vi "0006_FireAtSpecificTimeOnSpecificWeekdays.vi"(8 "error in (no error)":errorcluster) -> (0 "error out":errorcluster)   [LabVIEW 2013]
uses:
  <vilib>/addons/_JKI Toolkits/Caraya/classes/Assert/Assert True.vi
  <vilib>/addons/_JKI Toolkits/Caraya/classes/Test/Test.lvclass
  <vilib>/addons/_JKI Toolkits/Caraya/classes/Assert/Assert.lvclass
  source/openCron.lvlib
panel:
  out "after weekend":timestamp
  out "Occurences":timestamp[](array[timestamp])
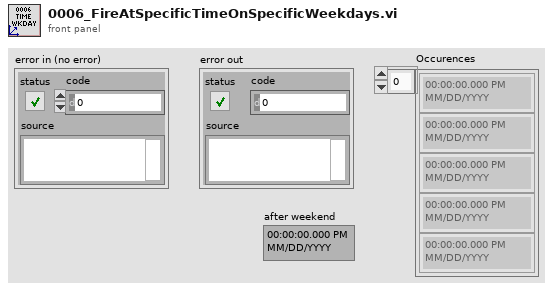
[diagram p1: front panel]
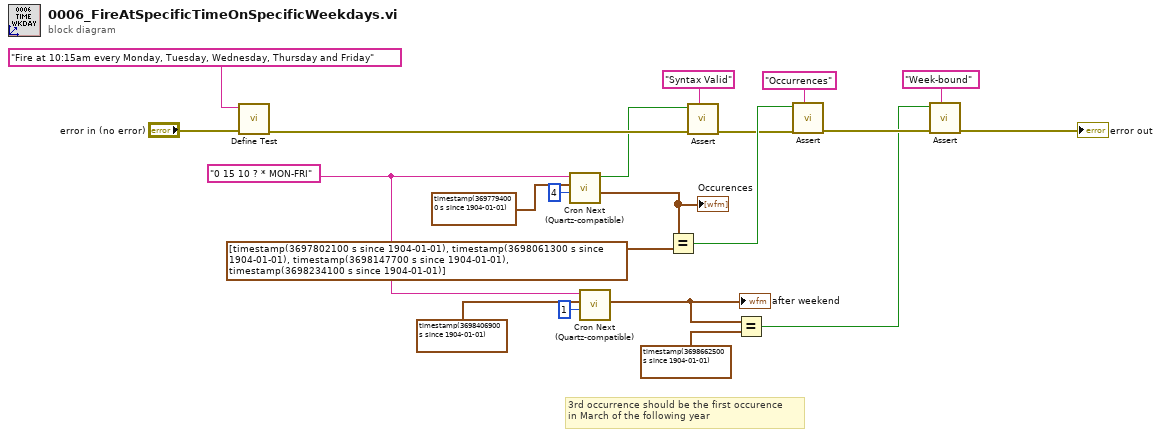
[diagram p0: block diagram]
diagram:
  w6 = "0 15 10 ? * MON-FRI" ("Expression")
  # "3rd occurrence should be the first occurence\nin March of the following year"
  n1 = call <vilib>:"Define Test.vi"("error in (no error)"="error in (no error)", "Label (VI Title)"="Fire at 10:15am every Monday, Tuesday, Wednesday, Thursday and Friday") -> ("error out"=w18:errorcluster)  [unwired: 9 in]
  n2 = call "Cron Next (Quartz-compatible).vi"("Nb Occurences (min: 1)"=u16 4, "Reference timestamp (Now)"=timestamp(3697794000 s since 1904-01-01) ("y"), "Cron Expression"=w6) -> ("Occurences"=w14:timestamp[], "syntax valid?"=w15:bool)  [unwired: 6 in, 1 out]
  "Occurences" <- w14
  n3 = call "Cron Next (Quartz-compatible).vi"("Nb Occurences (min: 1)"=u16 1, "Reference timestamp (Now)"=timestamp(3698406900 s since 1904-01-01) ("y"), "Cron Expression"=w6) -> ("Next Occurence"=w1:timestamp)  [unwired: 6 in, 2 out]
  "after weekend" <- w1
  n4 = Equal?(x=w14, y=timestamp[] [timestamp(3697802100 s since 1904-01-01), timestamp(3698061300 s since 1904-01-01), timestamp(3698147700 s since 1904-01-01), timestamp(3698234100 s since 1904-01-01)]) -> (x = y?=w17:bool)
  n5 = call-poly <vilib>:"Assert.vi"("Label"="Syntax Valid" ("Label (VI Title)"), "error in (no error)"=w18, "True?"=w15) -> ("error out"=w16:errorcluster)  [unwired: 8 in]
  n6 = Equal?(x=w1, y=timestamp(3698662500 s since 1904-01-01)) -> (x = y?=w3:bool)
  n7 = call-poly <vilib>:"Assert.vi"("Label"="Occurrences" ("Label (VI Title)"), "error in (no error)"=w16, "True?"=w17) -> ("error out"=w8:errorcluster)  [unwired: 8 in]
  n8 = call-poly <vilib>:"Assert.vi"("Label"="Week-bound" ("Label (VI Title)"), "error in (no error)"=w8, "True?"=w3) -> ("error out"=→"error out":errorcluster)  [unwired: 8 in]
